vi "Get Sensitivity.vi"(6 "sensitivity":sgl, 7 "pa":i32, 9 "amplifier":i32, 10 "horzShift":i32, 11 "channel":i32) -> (3 "function return":u32, 4 "sensitivity out":sgl)   [LabVIEW 2018, in "AndorSDK.lvlib"]
doc: "EXPNETTYPE unsigned int WINAPI GetSensitivity(int channel, int horzShift, int amplifier, int pa, float * sensitivity);"
uses:
  AndorSDK.lvlib
  ATMCD32D.dll
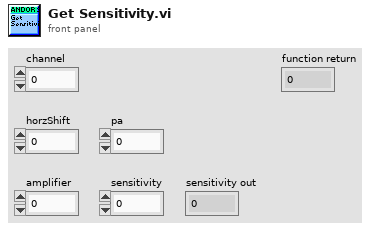
[diagram p1: front panel]
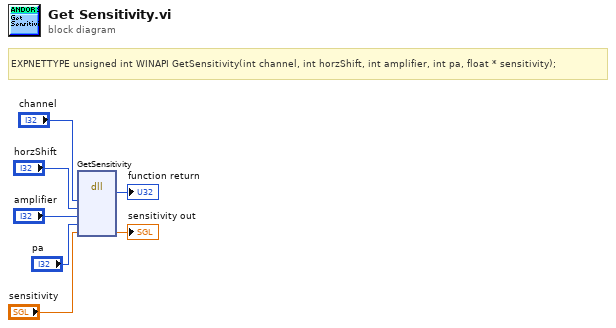
[diagram p0: block diagram]
diagram:
  # "EXPNETTYPE unsigned int WINAPI GetSensitivity(int channel, int horzShift, int amplifier, int pa, float * sensitivity);"
  n1 = dll-call lib="PTH2babs E\nPersönliches02 - Arbeit03-HiwijobsLabviewCodelibANDOR\tAndor SDK\nATMCD32D.*" fn="GetSensitivity"("channel"="channel", "horzShift"="horzShift", "amplifier"="amplifier", "pa"="pa", "sensitivity"="sensitivity") -> (→"function return":u32, "sensitivity"=→"sensitivity out":sgl)  [unwired: 7 in, 2 out]
